vi "WPI_Power Get PCM Compressor Current.vi"(0 "Pneumatics Control Module (0)":u8, 11 "error in":errorcluster) -> (6 "current (A)":dbl, 15 "error out":errorcluster)   [LabVIEW 2017]
doc: "Returns the current of the compressor on the Pneumatics Control Module (PCM)."
uses:
  <vilib>/Rock Robotics/WPI/CAN/PCM/WPI_CAN_PCMGlobalOps.ctl
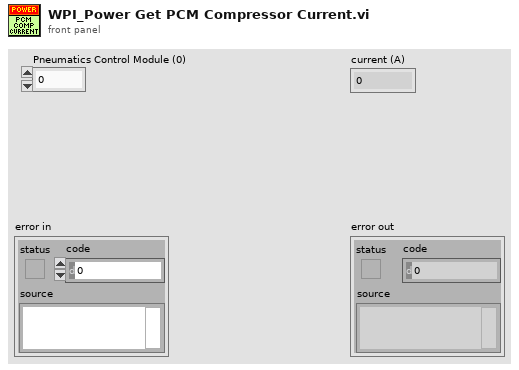
[diagram p1: front panel]
types:
  T1 = typedef "WPI_CAN_PCMGlobalOps.ctl" = enum16{"Read For Send", "Write After Receive", "Set Solenoids", "Set Closed Loop", "Clear Sticky Faults", "Get All", "Write Error", "Write After Receive Blacklist", "Set Control Frame Rate"}
  T2 = cluster{"Solenoid Status":bool[], "Battery Voltage":dbl, "Solenoid Voltage":dbl, "Compressor Current":dbl, "CompressorEnabled":bool, "StickySolenoidFault":bool, "StickyCompressorFault":bool, "SolenoidFault":bool, "CompressorFault":bool, "HardwareFault":bool, "ClosedLoopStatus":bool, "PressureStatus":bool, "Module Enabled":bool, "ClosedLoopSuggestedOutput":bool, "CAN Error":errorcluster, "Sticky Solenoid Faults":bool[]}
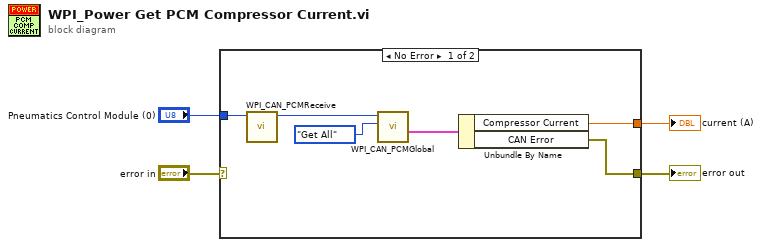
[diagram p0: block diagram]
diagram:
  n1 = case shown="No Error" "error in" {
    selector: "error in" -> [_ w11]
    tunnel: [w5 w11] -> w3
    tunnel: "Pneumatics Control Module (0)" -> [w6 _]
    tunnel: [w7 _] -> w1
    frame No Error {
      n2 = call <vilib>:"WPI_CAN_PCMReceive.vi"("Pneumatics Control Module (0)"=w6) -> ("Pneumatics Control Module Out"=w9:u8)  [unwired: 10 in]
      n3 = call <vilib>:"WPI_CAN_PCMGlobal.vi"("Operation"=WPI_CAN_PCMGlobalOps."Get All", "Pneumatics Control Module (0)"=w9) -> ("Get All"=w10:T2)  [unwired: 7 in, 2 out]
      n4 = Unbundle By Name(w10) -> ("Compressor Current"=w7:dbl, "CAN Error"=w5:errorcluster)
    }
    frame Error {
    }
  }
  "error out" <- w3
  "current (A)" <- w1
